vi "Merge Error.vi"(7 "Sender":refnum<class "Sender.lvclass">, 10 "Error":errorcluster, 11 "Base jettl in":refnum<class "Base jettl.lvclass">) -> (3 "Base jettl out":refnum<class "Base jettl.lvclass">)   [LabVIEW 2021, in "jettl.lvlib" / "Base jettl.lvclass"]
uses:
  Base jettl.lvclass
  Sender/Sender/Sender.lvclass
  Base jettl.lvclass/Base jettl.ctl
  State.ctl
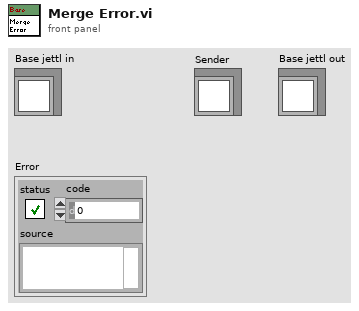
[diagram p1: front panel]
types:
  T1 = typedef "jettl.lvlib/Base jettl.lvclass/State.ctl" = enum16{"Nominal", "Teardown", "Error"}
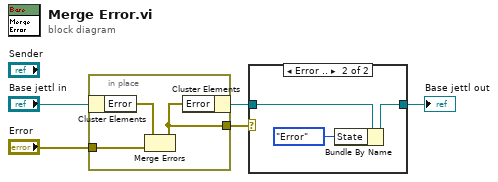
[diagram p0: block diagram]
diagram:
  n1 = in-place {
    in-place-border: "Error" -> [w7]
    in-place-border: [w6] -> w1
    n2 = in-place-cluster #1("Base jettl in") -> ("Error"=w8:errorcluster)
    n3 = Merge Errors(w8, w7) -> (w6:errorcluster)
    n4 = in-place-cluster #1("Error"=w6) -> (w3:refnum<class "Base jettl.lvclass">)
  }
  n5 = case shown="Error .." w1 {
    tunnel: [w9 w11] -> w2
    tunnel: w3 -> [w9 w12]
    frame No Error {
    }
    frame Error {
      n6 = Bundle By Name(cluster=w12, "State"=State."Error") -> (w11:refnum<class "Base jettl.lvclass">)
    }
  }
  "Base jettl out" <- w2
